vi "Get Compiled Settings.vi"(8 "error in":errorcluster, 11 "Variant":variant) -> (0 "error out":errorcluster, 3 "CompiledSettings":cluster{"Name":string})   [LabVIEW 2026, in "Template Debug Tools.lvlib"]
uses:
  Template Debug Tools.lvlib
  <vilib>/JDP Science/JSONtext/JSON text to Variant.vi
  <vilib>/Utility/Data Type/NI_Data Type.lvlib
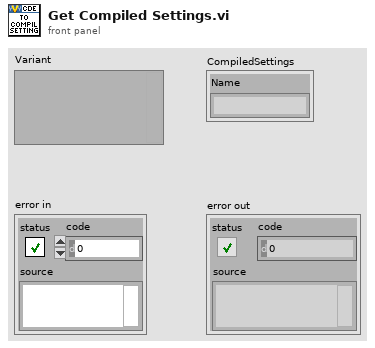
[diagram p1: front panel]
types:
  T1 = typedef "NI_Data Type.lvlib/Data Type.ctl" = enum8{"Invalid Type", "Void", "I8", "I16", "I32", "I64", "U8", "U16", "U32", "U64", "Single Float", "Double Float", "Extended Float", "Single Complex", "Double Complex", "Extended Complex", "Enum U8", "Enum U16", "Enum U32", "Enum U64", "Single Float With Unit", "Double Float With Unit", "Extended Float With Unit", "Single Complex with Unit", "Double Complex with Unit", "Extended Complex with Unit", "Boolean", "String", "Path", "Picture", "Tag", "Array", "Cluster", "Variant", "LV Variant", "Waveform", "Timestamp", "Digital Waveform", "Digital Data", "ExpressData", "Refnum", "External Data", "VI", "Poly VI", "LabVIEW Class Instance", "Fixed Point", "Set Collection", "Map Collection"}
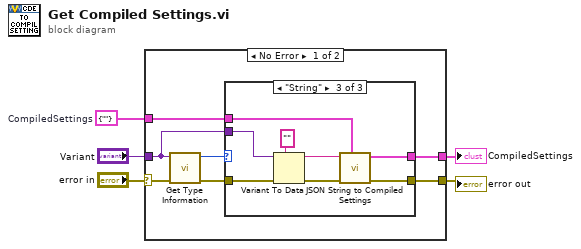
[diagram p0: block diagram]
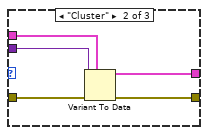
[diagram p3: hidden frame]
diagram:
  w3 = cluster{"Name":string} {"Name"=""}  # CompiledSettings
  n1 = case shown="No Error" "error in" {
    selector: "error in" -> [w12 w29]
    tunnel: "Variant" -> [w8 _]
    tunnel: w3 -> [w9 w28]
    tunnel: [w7 w29] -> w1
    tunnel: [w6 w28] -> w2
    frame No Error {
      n2 = call <vilib>:"Get Type Information.vi"("error in (no error)"=w12, "variant"=w8) -> ("error out"=w11:errorcluster, "type"=w10:T1)  [unwired: 5 in, 3 out]
      n3 = case shown="\"String\"" w10 {
        tunnel: w11 -> [w13 w19 w27]
        tunnel: w9 -> [w14 w18 w22]
        tunnel: w8 -> [_ w17 w26]
        tunnel: [w14 w16 w21] -> w6
        tunnel: [w13 w15 w20] -> w7
        frame Default {
        }
        frame "Cluster" {
          n4 = Variant To Data(error in=w19, type=w18, Variant=w17) -> (data=w16:cluster{"Name":string}, error out=w15:errorcluster)
        }
        frame "String" {
          n5 = Variant To Data(error in=w27, type="", Variant=w26) -> (data=w23:string, error out=w24:errorcluster)
          n6 = call "JSON String to Compiled Settings.vi"("CompiledSettings"=w22, "error in"=w24, "JSON"=w23) -> ("error out"=w20:errorcluster, "CompiledSettingsOut"=w21:cluster{"Name":string})  [unwired: 7 in]
        }
      }
    }
    frame Error {
    }
  }
  "CompiledSettings" <- w2
  "error out" <- w1
